vi "CRYGet Formated String Value.vi"(8 "Value":dbl, 11 "Flattened Format String":string) -> (3 "Unflattened Format string":string)   [LabVIEW 2013]
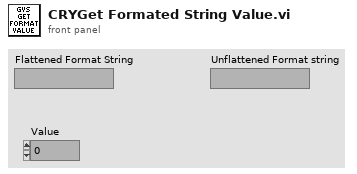
[diagram p1: front panel]
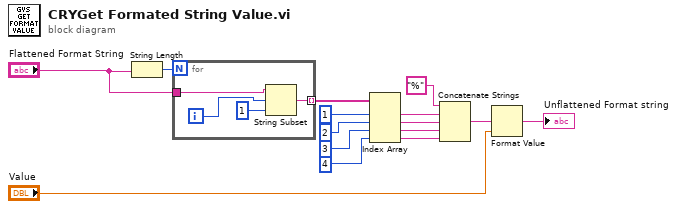
[diagram p0: block diagram]
diagram:
  n1 = String Length(string="Flattened Format String") -> (length=w10:i32)
  n2 = for {
    N: w10 -> [_]
    tunnel: "Flattened Format String" -> [w18]
    tunnel: [w16] -> w11 mode=indexing
    i -> [w17]
    n3 = String Subset(string=w18, offset (0)=w17, length (rest)=1 ("length (rest)")) -> (substring=w16:string)
  }
  n4 = Index Array(array=w11, index #1=1 ("index"), index #2=2 ("index"), index #3=3 ("index"), index #4=4 ("index")) -> (element #1=w9:string, element #2=w8:string, element #3=w7:string, element #4=w6:string)
  n5 = Concatenate Strings("%" ("string"), w9, w8, w7, w6) -> (w4:string)
  n6 = Format Value(format string=w4, value (0)="Value") -> (output string=→"Unflattened Format string":string)  [unwired: 1 in]
